vi "testing parse query string.vi"(11 "ENV":T1) -> (0 "Client Address":string, 2 "TestSeqId":string, 3 "Action":string)   [LabVIEW 2011]
uses:
  ITK EXT/utils/keyedarr.llb/Keyed Array.ctl
  ITK EXT/utils/strutil.llb/Case Matching.ctl
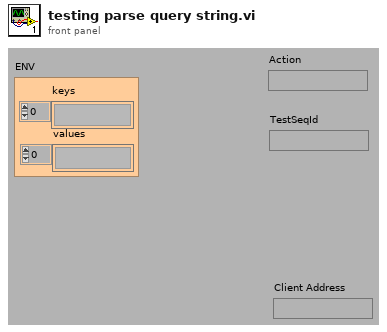
[diagram p1: front panel]
types:
  T1 = typedef "Keyed Array.ctl" = cluster{"keys":string[], "values":string[]}
  T2 = typedef "Case Matching.ctl" = enum16{"a != A", "a == A", "system"}
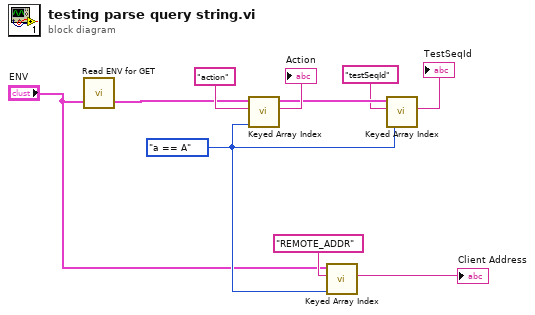
[diagram p0: block diagram]
diagram:
  w4 = Case_Matching."a == A" ("case matching (sensitive)")
  n1 = call "Read ENV for GET.vi"("ENV"="ENV") -> ("GET query params"=w1:T1)  [unwired: 2 out]
  n2 = call "Keyed Array Index.vi"("case matching (sensitive)"=w4, "key"="action", "array in"=w1) -> ("value"=→"Action":string, "duplicate array"=w8:T1)  [unwired: 1 in, 2 out]
  n3 = call "Keyed Array Index.vi"("case matching (sensitive)"=w4, "key"="REMOTE_ADDR", "array in"="ENV") -> ("value"=→"Client Address":string)  [unwired: 1 in, 3 out]
  n4 = call "Keyed Array Index.vi"("case matching (sensitive)"=w4, "key"="testSeqId", "array in"=w8) -> ("value"=→"TestSeqId":string)  [unwired: 1 in, 3 out]
